vi "delay_selector.vi"(2 "Delay in":dbl format="%#_13g", 3 "T1":dbl format="%#_13g") -> (7 "Delay out":dbl)   [LabVIEW 2015]
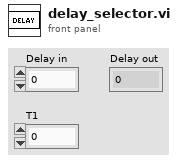
[diagram p1: front panel]
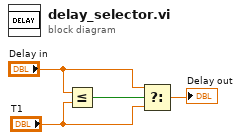
[diagram p0: block diagram]
diagram:
  n1 = Less Or Equal?(x="Delay in", y="T1") -> (x <= y?=w1:bool)
  n2 = Select(t="Delay in", s=w1, f="T1") -> (s? t:f=→"Delay out":dbl)
